vi "Set Frequency and Phase.vi"(5 "CS Channel":u8, 6 "Ref Clock Freq (125MHz)":dbl=125000000.0 format="%#_6p", 7 "SPI Channel (0)":u8, 8 "Error In":errorcluster, 9 "Phase Offset (5-bit)":u8, 10 "Frequency":u32, 11 "LINX Resource":T1) -> (0 "Error Out":errorcluster, 3 "LINX Resource":T1)   [LabVIEW 2020, in "LMH-LINX.lvlib" / "AD9850.lvlib"]
doc: "Set the frequency and phase of the AD9850 output signal."
uses:
  AD9850.lvlib
  Private/Type Defs/LINX Ref.ctl
  Private/Type Defs/Platform.ctl
  Private/Device/Type Defs/LINX Device Config.ctl
  Private/Type Defs/Interface.ctl
  Private/Device/Type Defs/TCP Config.ctl
  Private/Device/Type Defs/Channels.ctl
  Peripherals/SPI/SPI CS Config.ctl
  Private/Type Defs/Peripherals/SPI/SPI CS Logic Level.ctl
  Peripherals/SPI/SPI Write Read 1 Frame.vi
  Peripherals/SPI/SPI Write Read N Frames.vi
  Private/Local IO/LinxSpiWriteRead.vi
  Utilities/Check Channel.vi
  Private/Utilties/Generate Error.vi
  LMH-LINX.lvlib
  Private/Device/Device.lvlib
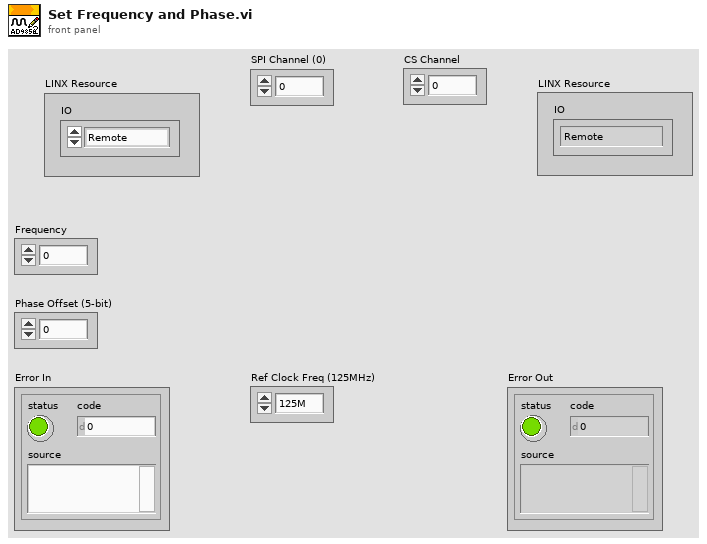
[diagram p1: front panel]
types:
  T1 = typedef "LMH-LINX.lvlib/LINX Ref.ctl" = cluster{"IO":T2, "LINX Device Config":T3}
  T2 = typedef "LMH-LINX.lvlib/Platform.ctl" = enum16{"Remote", "Local"}
  T3 = typedef "Device.lvlib/LINX Device Config.ctl" = cluster{"Interface":T4, "COM Port":refnum<visa-resource-name>, "TCP Configuration":T5, "Device Family":u8, "Device ID":u8, "Device Name":string, "TCP Ref":refnum<k5>, "Local Refnum":u64, "Channels":T6}
  T4 = typedef "LMH-LINX.lvlib/Interface.ctl" = enum16{"Serial", "TCP"}
  T5 = typedef "Device.lvlib/TCP Config.ctl" = cluster{"IP Address":string, "Port":u16}
  T6 = typedef "LMH-LINX.lvlib/Channels.ctl" = cluster{"DI":u8[], "DO":u8[], "AI":u8[], "AO":u8[], "PWM":u8[], "QE":u8[], "UART":u8[], "I2C 2":u8[], "SPI":u8[], "CAN":u8[], "Servo":u8[], "AI Ref (V)":dbl, "AI Resolution (Bits)":u8, "AO Ref (V)":dbl, "AO Resolution (Bits)":u8}
  T7 = typedef "LMH-LINX.lvlib/SPI CS Config.ctl" = cluster{"CS Channel":u8, "CS Logic Level":T8}
  T8 = typedef "LMH-LINX.lvlib/SPI CS Logic Level.ctl" = enum8{"Active Low", "Active High"}
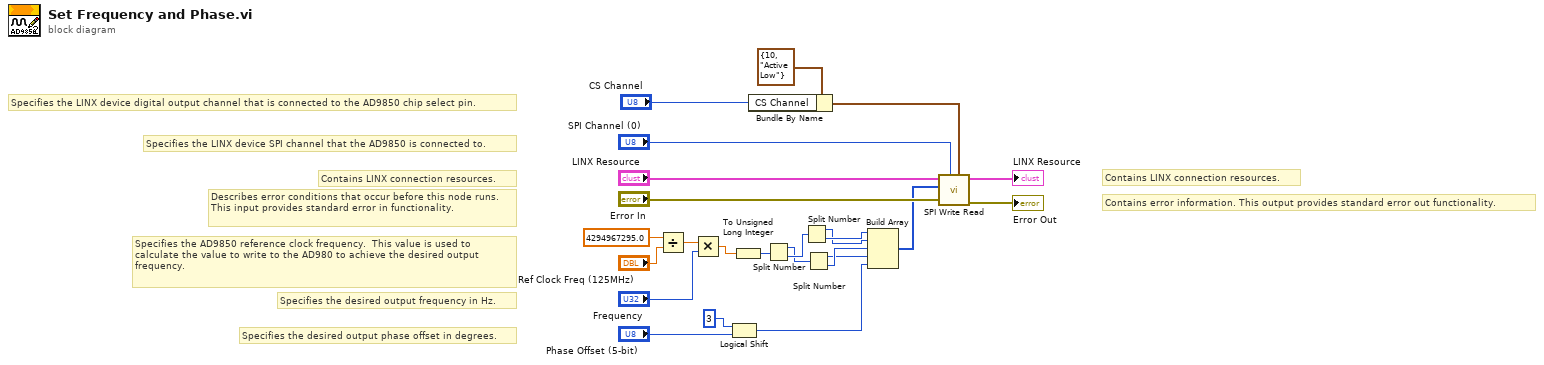
[diagram p0: block diagram]
diagram:
  # "Specifies the desired output phase offset in degrees."
  # "Specifies the desired output frequency in Hz."
  # "Specifies the AD9850 reference clock frequency.  This value is used to calculate the value to write to the AD980 to achieve the desired output frequency."
  # "Specifies the LINX device SPI channel that the AD9850 is connected to."
  # "Specifies the LINX device digital output channel that is connected to the AD9850 chip select pin."
  # "Contains LINX connection resources."
  # "Contains error information. This output provides standard error out functionality."
  # "Contains LINX connection resources."
  # "Describes error conditions that occur before this node runs. This input provides standard error in functionality."
  n1 = Divide(x=4294967295.0, y="Ref Clock Freq (125MHz)") -> (x/y=w18:dbl)
  n2 = Multiply(x=w18, y="Frequency") -> (x*y=w12:dbl)
  n3 = Logical Shift(y=i8 3, x="Phase Offset (5-bit)") -> (x << y=w10:u8)
  n4 = To Unsigned Long Integer(number=w12) -> (unsigned 32bit integer=w11:u32)
  n5 = Bundle By Name(cluster=T7 {"CS Channel"=10, "CS Logic Level"=enum."Active Low"} ("CS Configuration"), "CS Channel"="CS Channel") -> (w1:T7)
  n6 = Split Number(x=w11) -> (hi(x)=w19:u16, lo(x)=w20:u16)
  n7 = Split Number(x=w20) -> (hi(x)=w23:u8, lo(x)=w24:u8)
  n8 = Split Number(x=w19) -> (hi(x)=w21:u8, lo(x)=w22:u8)
  n9 = Build Array(w24, w23, w22, w21, w10) -> (w5:u8[])
  n10 = call-poly "SPI Write Read.vi"("CS Configuration"=w1, "SPI Channel (0)"="SPI Channel (0)", "Error In"="Error In", "Data"=w5, "LINX Resource"="LINX Resource") -> ("Error Out"=→"Error Out":errorcluster, "LINX Resource"=→"LINX Resource":T1)  [unwired: 3 in, 2 out]
